vi "IO@CheckLogicOff__Parameter.vi"(1 "ParamterIn":string) -> (0 "ParamterOut":string)   [LabVIEW 2020]
panel:
  in  "Confirm":bool
  in  "Message":string(combo)
  in  "TimeOut":string(combo)
  in  "PortSelect":string(combo)
  # "IO@CheckLogicOff $IOLogic(,$Timeout,[[$label]]$Message)\nIOLogic Express is:\nIO1 & (IO2 | IO3)\nVar==XXX, !=XXX, >=XXX, <=XXX, >XXX, <XXX\nVar <> XXX~YYY, </>XXX~YYY\nVar==NULL, ==EXIST, ==[], ==[;;]\nVar !=NULL, !=EXIST, !=[], !=[;;]\n~IOLogic will inverse Logic\nUse Var@Section to assign which section"
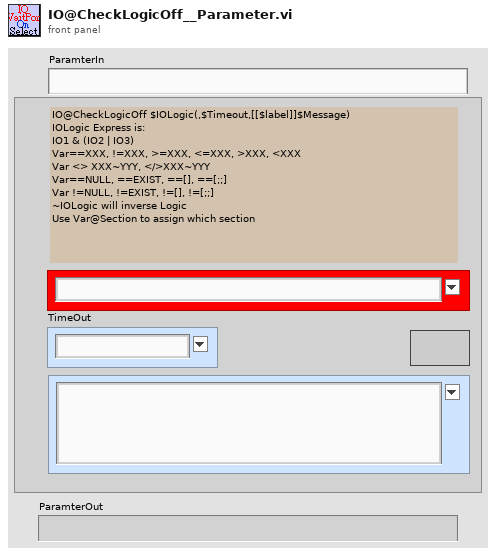
[diagram p1: front panel]
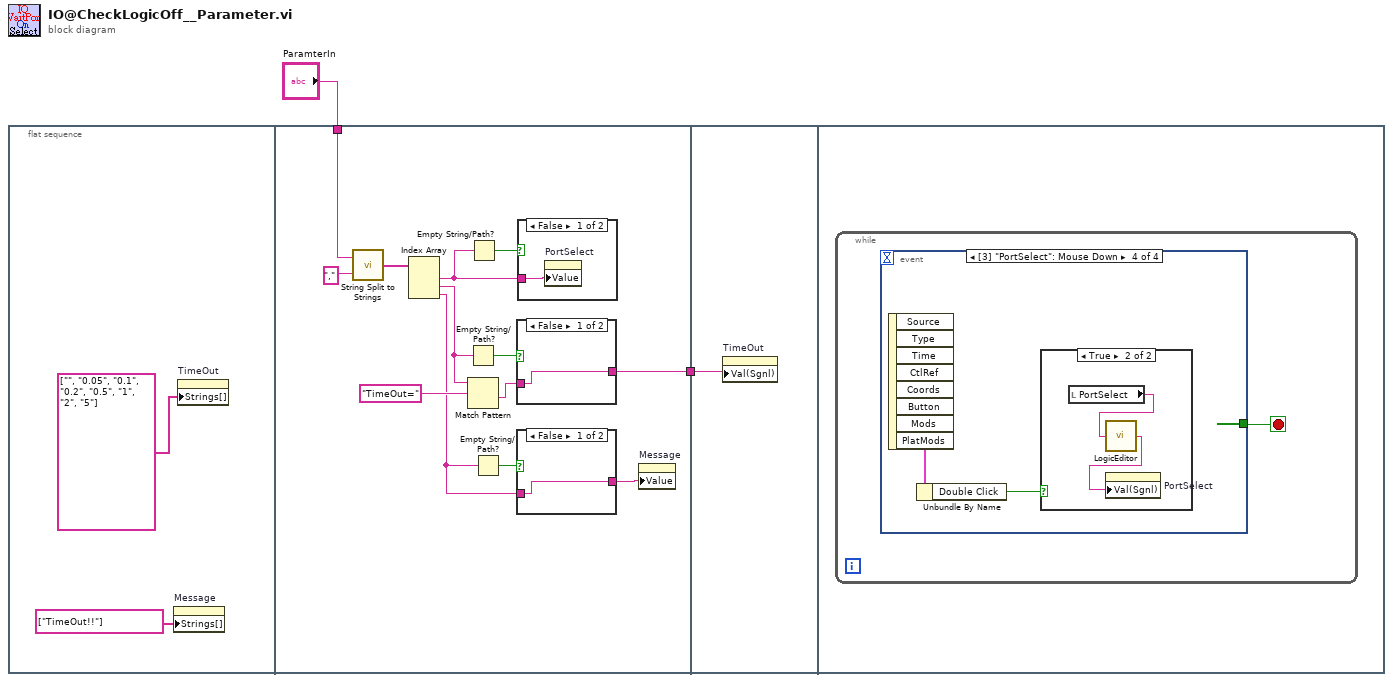
[diagram p0: block diagram]
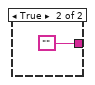
[diagram p2: hidden frame]
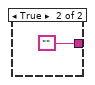
[diagram p3: hidden frame]
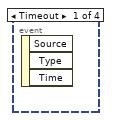
[diagram p5: hidden frame]
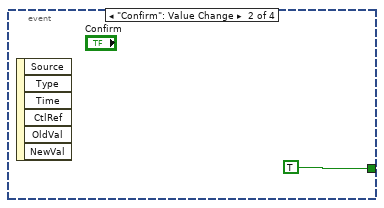
[diagram p6: hidden frame]
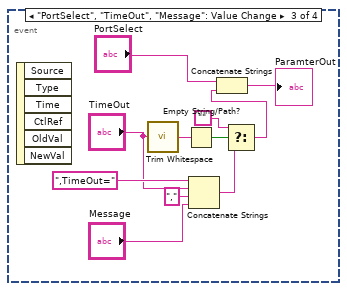
[diagram p7: hidden frame]
diagram:
  n1 = flat-sequence {
    tunnel: "ParamterIn" -> [w16]
    tunnel: [w8] -> w1
    tunnel: w1 -> [w23]
    frame #0 {
      n2 = property on="Message" class="CmbBox"("Strings[]"=string[] ["TimeOut!!"] ("Strings []")) -> ()  [unwired: 2 in, 2 out]
      n3 = property on="TimeOut" class="CmbBox"("Strings[]"=string[] ["", "0.05", "0.1", "0.2", "0.5", "1", "2", "5"] ("Strings []")) -> ()  [unwired: 2 in, 2 out]
    }
    frame #1 {
      n4 = call "String Split to Strings.vi"("search string/char (-)"=",", "String"=w16) -> ("Array"=w15:string[])
      n5 = Index Array(array=w15) -> (element #1=w13:string, element #2=w10:string, element #3=w6:string)  [unwired: 3 in]
      n6 = Empty String/Path?(string/path=w10) -> (empty?=w12:bool)
      n7 = Match Pattern(string=w10, regular expression="TimeOut=") -> (after substring=w11:string)  [unwired: 1 in, 3 out]
      n8 = Empty String/Path?(string/path=w13) -> (empty?=w14:bool)
      n9 = Empty String/Path?(string/path=w6) -> (empty?=w7:bool)
      n10 = case shown="False" w12 {
        tunnel: w11 -> [w20 _]
        tunnel: [w20 ""] -> w8
        frame False {
        }
        frame True {
        }
      }
      n11 = case shown="False" w7 {
        tunnel: w6 -> [w18 _]
        tunnel: [w18 ""] -> w5
        frame False {
        }
        frame True {
        }
      }
      n12 = case shown="False" w14 {
        tunnel: w13 -> [w22 _]
        frame False {
          n13 = property on="PortSelect" class="CmbBox"("Value"=w22) -> ()  [unwired: 2 in, 2 out]
        }
        frame True {
        }
      }
      n14 = property on="Message" class="CmbBox"("Value"=w5) -> ()  [unwired: 2 in, 2 out]
    }
    frame #2 {
      n15 = property on="TimeOut" class="CmbBox"("Val(Sgnl)"=w23) -> ()  [unwired: 2 in, 2 out]
    }
    frame #3 {
      n16 = while {
        stop <- w24 stop-if-true
        n17 = event shown="[3] \"PortSelect\": Mouse Down" {
          selector: _ -> [_ _ _ _]
          dyn-events: _ -> [_ _ _ _]
          timeout: _ -> [_ _ _ _]
          tunnel: [_ TRUE _ _] -> w24
          event Timeout {
            n18 = event-data() -> ()  [unwired: 1 in, 3 out]
          }
          event "Confirm": Value Change {
            n19 = event-data() -> ()  [unwired: 1 in, 6 out]
          }
          event "PortSelect", "TimeOut", "Message": Value Change {
            n20 = event-data() -> ()  [unwired: 1 in, 6 out]
            n21 = call <vilib>:"Trim Whitespace.vi"("string"="TimeOut") -> ("trimmed string"=w30:string)  [unwired: 1 in]
            n22 = Empty String/Path?(string/path=w30) -> (empty?=w31:bool)
            n23 = Concatenate Strings(",TimeOut=" ("string"), "TimeOut", "," ("string"), "Message") -> (w33:string)
            n24 = Select(t="", s=w31, f=w33) -> (s? t:f=w28:string)
            n25 = Concatenate Strings("PortSelect", w28) -> (→"ParamterOut":string)
          }
          event "PortSelect": Mouse Down {
            n26 = event-data() -> ("Mods"=w38:cluster{"Double Click":bool, "Menu Key":bool})  [unwired: 1 in, 7 out]
            n27 = Unbundle By Name(w38) -> ("Double Click"=w37:bool)
            n28 = case shown="True" w37 {
              frame False {
              }
              frame True {
                n29 = local read "PortSelect"() -> (w40:string)
                n30 = call "LogicEditor.vi"("Logic Express"=w40) -> ("LogicExpressOut"=w39:string)
                n31 = property on="PortSelect" class="CmbBox"("Val(Sgnl)"=w39) -> ()  [unwired: 2 in, 2 out]
              }
            }
          }
        }
      }
    }
  }
